vi "Auto Setup.vi"(8 "error in":errorcluster) -> (0 "error out":errorcluster)   [LabVIEW 2020]
uses:
  <vilib>/Rock Robotics/WPI/DriverStation/WPI_DriverStationRobotMode2.ctl
  b3a484b6-3d34-4235-842a-44c07264b682.vi
  19e807a5-ee4b-41d9-ac37-e9a2df102fa4.vi
  Framework/Robot Global Data.vi
  <vilib>/Rock Robotics/Network Tables/NT Write String Array.vi
  <vilib>/Rock Robotics/Network Tables/NT Write Variant.vi
panel:
  in  "override":bool=TRUE
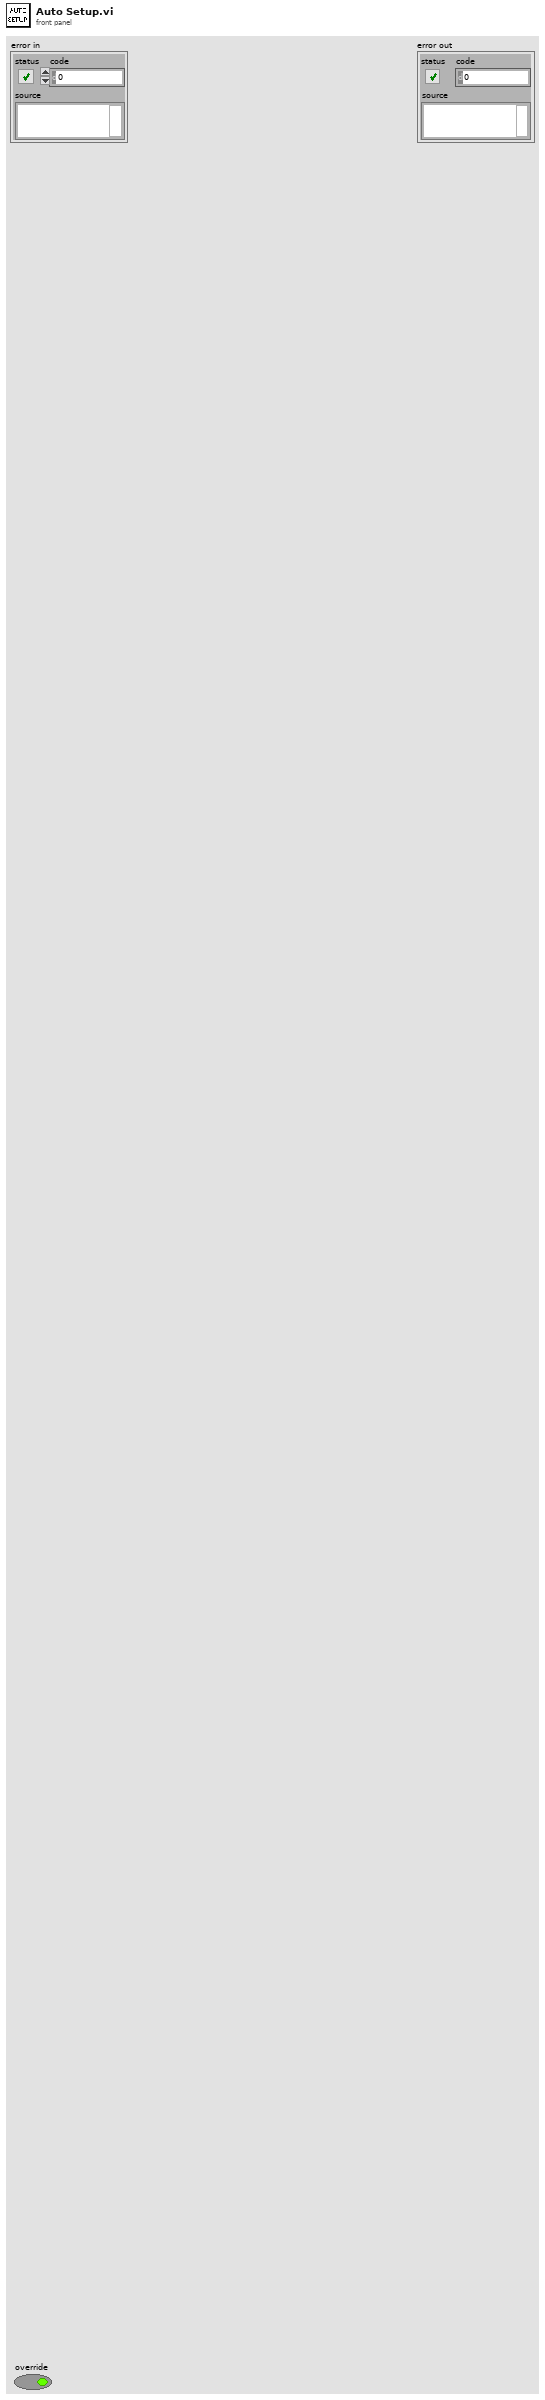
[diagram p1: front panel]
types:
  T1 = typedef "WPI_DriverStationRobotMode2.ctl" = enum16{"Autonomous Disabled", "Autonomous Enabled", "Teleop Disabled", "Teleop Enabled", "Disconnected", "Finish", "Test Disabled", "Test Enabled", "Emergency Stopped"}
  T2 = cluster{"Robot Backwards":bool, "Reverse Path":bool}
  T3 = cluster{"Segment Name":string, "Type":enum16{"Accel Straight", "Const Straight", "Blend", "Circle"}, "Traj Pos Points":cluster{"x":dbl, "y":dbl, "th":dbl}[], "Traj Vel Points":cluster{"V":dbl, "th":dbl}[], "Accel Index":i32, "Decel Index":i32}[]
  T4 = typedef "Single Cmd Info.ctl" = cluster{"Name":string, "CPTM.DataType":variant, "All Control Values Variant":cluster{"Name":string, "Variant Data":variant}[], "icon full":T5, "icon scaled":T5, "Path":path, "Subsystem Color":u32}
  T5 = typedef "imagedata.ctl" = cluster{"image type":i32, "image depth":i32, "image":u8[], "mask":u8[], "colors":u32[], "Rectangle":cluster{"left":i16, "top":i16, "right":i16, "bottom":i16}}
  T6 = typedef "Overrides.ctl" = cluster{"Count":string, "Angular Override":dbl, "Enabled?":bool, "Velocity Override":dbl, "Angle Override":dbl}[]
  T7 = typedef "Angluar Limits.ctl" = cluster{"Velocity (deg/s)":dbl, "Accel (deg/s^2)":dbl, "Jerk (deg/s^3)":dbl}
  T8 = cluster{"Sample Period (s)":dbl, cluster{"Velocity (fps)":dbl, "Accel (fps^2)":dbl, "Jerk (fps^3)":dbl, "StoopidFast (fps)":dbl}, "Conditions":cluster{"vInitial (fps)":dbl, "vFinal (fps)":dbl}, "Overrides":T6, "Angular Limits":T7}
  T9 = typedef "Drive Type.ctl" = enum16{"Nonholonomic", "Holonomic"}
  T10 = typedef "Path Type.ctl" = enum16{"Clothoid", "Bezier"}
  T11 = cluster{"Overall":cluster{"Time (s)":dbl, "Distance (ft)":dbl}, "Points out":cluster{"x":dbl, "y":dbl, "th":dbl}[], "Commands out":cluster{"Time (s)":dbl, T4, bool}[], "Zero V":bool, "Trajectory Data":cluster{"Segment Name":string, "Type":enum16{"Accel Straight", "Const Straight", "Blend", "Circle"}, "Traj Pos Points":cluster{"x":dbl, "y":dbl, "th":dbl}[], "Traj Vel Points":cluster{"V":dbl, "th":dbl}[], "Accel Index":i32, "Decel Index":i32}[], "Reversals":cluster{"Robot Backwards":bool, "Reverse Path":bool}, "Fields":cluster{"Sample Period (s)":dbl, cluster{"Velocity (fps)":dbl, "Accel (fps^2)":dbl, "Jerk (fps^3)":dbl, "StoopidFast (fps)":dbl}, "Conditions":cluster{"vInitial (fps)":dbl, "vFinal (fps)":dbl}, "Overrides":T6, "Angular Limits":T7}, "Trajectory Meta":cluster{"Drive Type":T9, "Path Type":T10}}
  T12 = cluster{"Traj Vel Points":cluster{"V":dbl, "th":dbl}[], "Reversals":cluster{"Robot Backwards":bool, "Reverse Path":bool}}
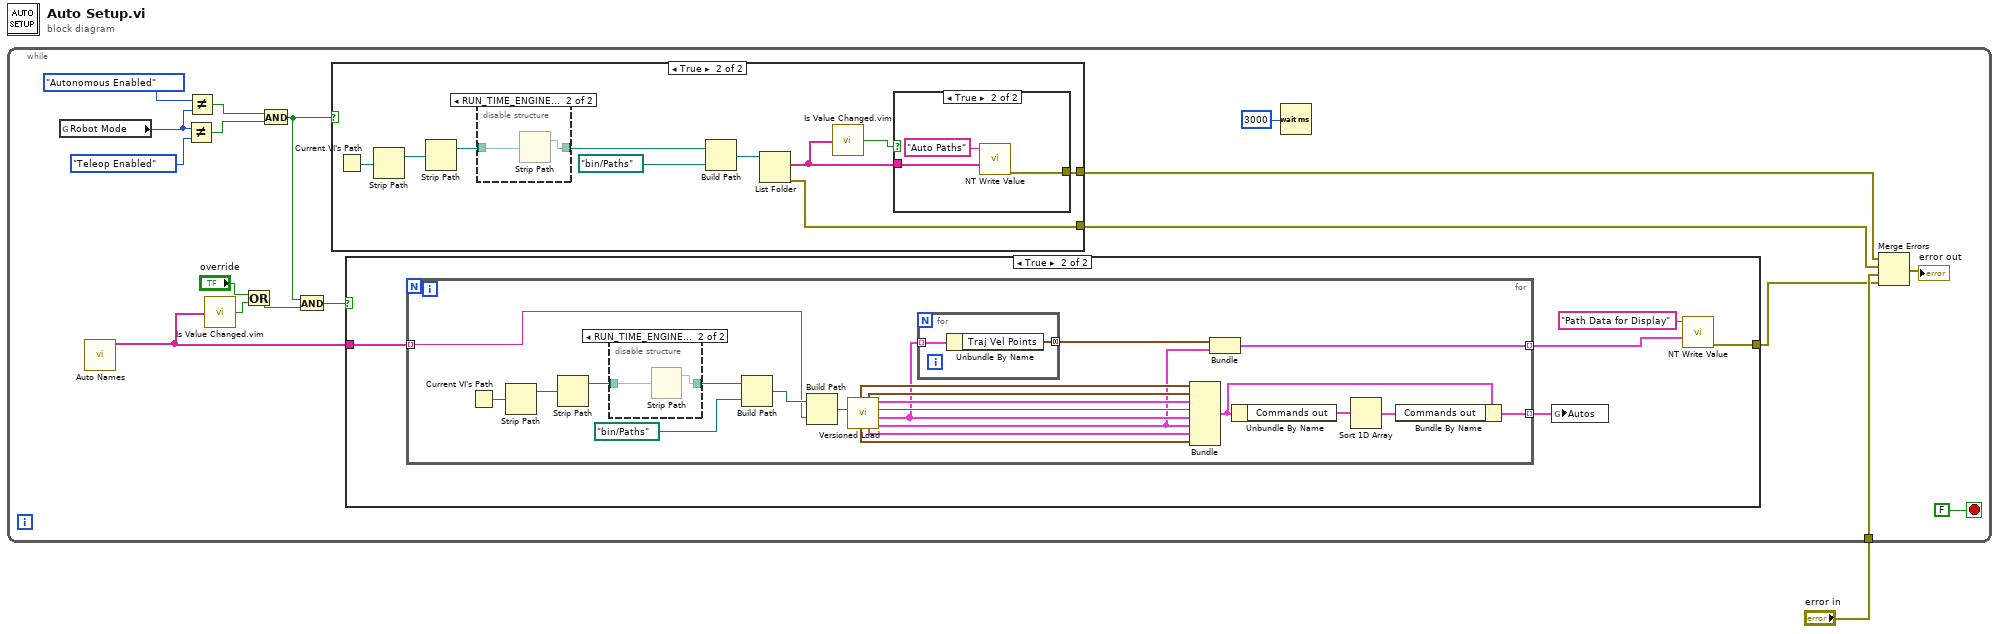
[diagram p0: block diagram]
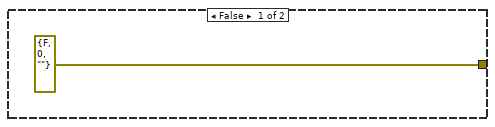
[diagram p2: hidden frame]
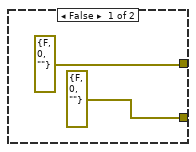
[diagram p4: hidden frame]
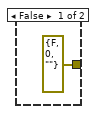
[diagram p5: hidden frame]
diagram:
  n1 = while {
    tunnel: "error in" -> [w4]
    stop <- FALSE stop-if-true
    n2 = global read "Robot Global Data.vi" "Robot Mode"() -> (w17:T1)
    n3 = call "Auto Names.vi"() -> ("Path Names"=w2:string[])  [unwired: 11 in]
    n4 = Not Equal?(x=w17, y=WPI_DriverStationRobotMode2."Teleop Enabled") -> (x != y?=w14:bool)
    n5 = Not Equal?(x=WPI_DriverStationRobotMode2."Autonomous Enabled", y=w17) -> (x != y?=w15:bool)
    n6 = call "Is Value Changed.vim"("value"=w2) -> ("changed or first call?"=w8:bool)
    n7 = Or(x="override", y=w8) -> (x .or. y?=w6:bool)
    n8 = And(x=w15, y=w14) -> (x .and. y?=w5:bool)
    n9 = And(x=w5, y=w6) -> (x .and. y?=w13:bool)
    n10 = case shown="True" w5 {
      tunnel: [errorcluster {"status"=FALSE, "code"=0, "source"=""} ("error out") w58] -> w12
      tunnel: [errorcluster {"status"=FALSE, "code"=0, "source"=""} ("error out") w57] -> w10
      frame False {
      }
      frame True {
        n11 = Current VI's Path() -> (path=w60:path)
        n12 = Strip Path(path=w60) -> (stripped path=w61:path)  [unwired: 1 out]
        n13 = Strip Path(path=w61) -> (stripped path=w63:path)  [unwired: 1 out]
        n14 = disable-structure shown="RUN_TIME_ENGINE==True, Default" {
          disable-tunnel: [w69 w70] -> w62
          disable-tunnel: w63 -> [w69 w71]
          frame condition #0 (active) {
          }
          frame condition #1 {
            n15 = Strip Path(path=w71) -> (stripped path=w70:path)  [unwired: 1 out]
          }
        }
        n16 = Build Path(base path=w62, name or relative path=path "bin/Paths") -> (appended path=w64:path)
        n17 = List Folder(path=w64) -> (filenames=w56:string[], error out=w58:errorcluster)  [unwired: 3 in, 2 out]
        n18 = call "Is Value Changed.vim"("value"=w56) -> ("changed or first call?"=w55:bool)
        n19 = case shown="True" w55 {
          tunnel: w56 -> [_ w67]
          tunnel: [errorcluster {"status"=FALSE, "code"=0, "source"=""} ("error out") w66] -> w57
          frame False {
          }
          frame True {
            n20 = call-poly <vilib>:"NT Write Value.vi"("String Array"=w67, "Name"="Auto Paths") -> ("error out"=w66:errorcluster)  [unwired: 9 in]
          }
        }
      }
    }
    n21 = case shown="True" w13 {
      tunnel: w2 -> [_ w23]
      tunnel: [errorcluster {"status"=FALSE, "code"=0, "source"=""} ("error out") w24] -> w3
      frame False {
      }
      frame True {
        n22 = for {
          tunnel: w23 -> [w41] mode=indexing
          tunnel: [w40] -> w22 mode=indexing
          tunnel: [w28] -> w21 mode=indexing
          n23 = Current VI's Path() -> (path=w47:path)
          n24 = Strip Path(path=w47) -> (stripped path=w46:path)  [unwired: 1 out]
          n25 = Strip Path(path=w46) -> (stripped path=w44:path)  [unwired: 1 out]
          n26 = disable-structure shown="RUN_TIME_ENGINE==True, Default" {
            disable-tunnel: [w50 w51] -> w45
            disable-tunnel: w44 -> [w50 w52]
            frame condition #0 (active) {
            }
            frame condition #1 {
              n27 = Strip Path(path=w52) -> (stripped path=w51:path)  [unwired: 1 out]
            }
          }
          n28 = Build Path(base path=w45, name or relative path=path "bin/Paths") -> (appended path=w42:path)
          n29 = Build Path(base path=w42, name or relative path=w41) -> (appended path=w39:path)
          n30 = call "Versioned Load.vi"("path"=w39) -> ("Reversals"=w30:T2, "Trajectory Data"=w33:T3, "Zero V"=w34:bool, "Commands out"=w35:cluster{"Time (s)":dbl, T4, bool}[], "Fields"=w32:T8, "Points out"=w36:cluster{"x":dbl, "y":dbl, "th":dbl}[], "Trajectory Meta"=w31:cluster{"Drive Type":T9, "Path Type":T10}, "Overall"=w37:cluster{"Time (s)":dbl, "Distance (ft)":dbl})  [unwired: 3 in]
          n31 = for {
            tunnel: w33 -> [w49] mode=indexing
            tunnel: [w48] -> w38 mode=concatenating
            n32 = Unbundle By Name(w49) -> ("Traj Vel Points"=w48:cluster{"V":dbl, "th":dbl}[])
          }
          n33 = Bundle("Overall"=w37, "Points out"=w36, "Commands out"=w35, "Zero V"=w34, "Trajectory Data"=w33, "Reversals"=w30, "Fields"=w32, "Trajectory Meta"=w31) -> (w29:T11)  [unwired: 1 in]
          n34 = Bundle("Traj Vel Points"=w38, "Reversals"=w30) -> (w40:T12)  [unwired: 1 in]
          n35 = Unbundle By Name(w29) -> ("Commands out"=w27:cluster{"Time (s)":dbl, T4, bool}[])
          n36 = Sort 1D Array(array=w27) -> (sorted array=w26:cluster{"Time (s)":dbl, T4, bool}[])
          n37 = Bundle By Name(cluster=w29, "Commands out"=w26) -> (w28:T11)
        }
        n38 = global write "Robot Global Data.vi" "Autos"(w21) -> ()
        n39 = call-poly <vilib>:"NT Write Value.vi"("Variant"=w22, "Name"="Path Data for Display") -> ("error out"=w24:errorcluster)  [unwired: 9 in]
      }
    }
    n40 = Wait (ms)(milliseconds to wait=u32 3000) -> ()  [unwired: 1 out]
    n41 = Merge Errors(w10, w12, w4, w3) -> (→"error out":errorcluster)
  }
